vi "Crop camera.vi"(6 "error in (no error)":errorcluster, 7 "Cropping":T1={"PosX"=0, "PosY"=0, "Height"=2054, "Width"=2456} {"Width" min=0 max=1956 step=1; "Height" min=0 max=2054 step=1; "PosY" min=0 max=0 step=1; "PosX" min=0 max=2336 step=1}, 9 ".NET Refnum in":refnum<k24>) -> (0 "error out":errorcluster, 3 ".NET Refnum out":refnum<k24>)   [LabVIEW 2017]
uses:
  C:/Program Files/National Instruments/LabVIEW 2017/instr.lib/IDS/ueye.NET/uEyeDotNet.dll
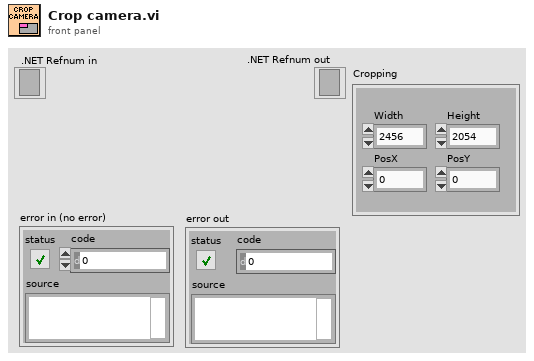
[diagram p1: front panel]
types:
  T1 = cluster{"PosX":i32, "PosY":i32, "Height":i32, "Width":i32}
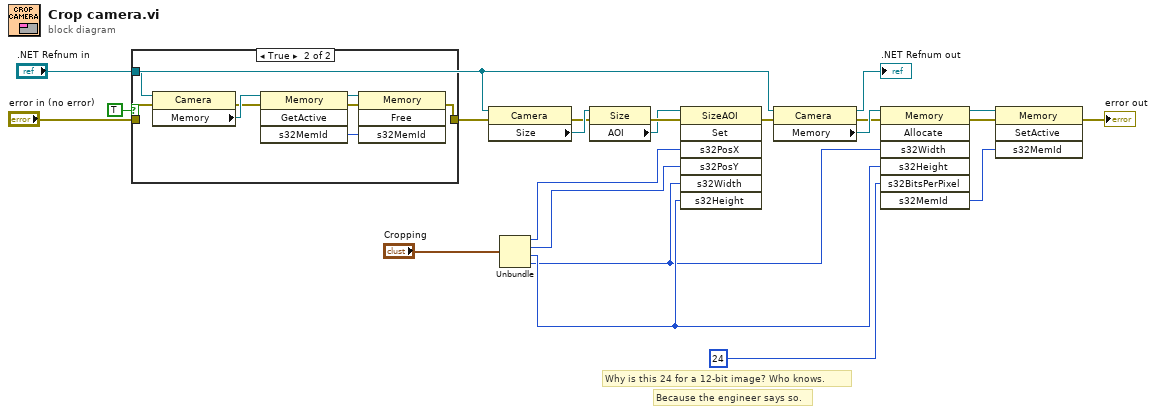
[diagram p0: block diagram]
diagram:
  # "Because the engineer says so."
  # "Why is this 24 for a 12-bit image? Who knows."
  n1 = case shown="True" TRUE {
    tunnel: "error in (no error)" -> [w23 w27]
    tunnel: ".NET Refnum in" -> [_ w25]
    tunnel: [w23 w24] -> w7
    frame False {
    }
    frame True {
      n2 = property class="Camera"(reference=w25, error in=w27) -> (error out=w26:errorcluster, "Memory"=w31:refnum<k24>)  [unwired: 1 out]
      n3 = invoke class="Memory" method="GetActive"(reference=w31, error in=w26) -> (reference out=w30:refnum<k24>, error out=w29:errorcluster, "s32MemId"=w28:i32)  [unwired: 2 in, 1 out]
      n4 = invoke class="Memory" method="Free"(reference=w30, error in=w29, "s32MemId"=w28) -> (error out=w24:errorcluster)  [unwired: 1 in, 3 out]
    }
  }
  n5 = property class="Camera"(reference=".NET Refnum in", error in=w7) -> (error out=w16:errorcluster, "Size"=w17:refnum<k24>)  [unwired: 1 out]
  n6 = Unbundle("Cropping") -> ("PosX"=w5:i32, "PosY"=w4:i32, "Height"=w3:i32, "Width"=w2:i32)
  n7 = property class="Size"(reference=w17, error in=w16) -> (error out=w19:errorcluster, "AOI"=w18:refnum<k24>)  [unwired: 1 out]
  n8 = invoke class="SizeAOI" method="Set"(reference=w18, error in=w19, "s32PosX"=w5, "s32PosY"=w4, "s32Width"=w2, "s32Height"=w3) -> (error out=w15:errorcluster)  [unwired: 1 in, 6 out]
  n9 = property class="Camera"(reference=".NET Refnum in", error in=w15) -> (reference out=→".NET Refnum out":refnum<k24>, error out=w14:errorcluster, "Memory"=w21:refnum<k24>)
  n10 = invoke class="Memory" method="Allocate"(reference=w21, error in=w14, "s32Width"=w2, "s32Height"=w3, "s32BitsPerPixel"=24) -> (reference out=w11:refnum<k24>, error out=w13:errorcluster, "s32MemId"=w10:i32)  [unwired: 2 in, 4 out]
  n11 = invoke class="Memory" method="SetActive"(reference=w11, error in=w13, "s32MemId"=w10) -> (error out=→"error out":errorcluster)  [unwired: 1 in, 3 out]
